vi "3d queue - Copia.vi"() -> ()   [LabVIEW 2020]
uses:
  control/Data Form.ctl
  control/file structure.ctl
  <vilib>/Analysis/1siggen.llb/Ramp Pattern by Samples.vi
  queue/Front Panel Message Queue.lvlib
  <vilib>/Analysis/NI_AALBase.lvlib
panel:
  out "XY Graph":cluster{"Ramp Pattern":dbl[], dbl[]}(graph)
  out "Data Loaded":dbl[][](array[numeric])
  out "Data Form":T1
  out "error out":errorcluster
  in  "error in":errorcluster
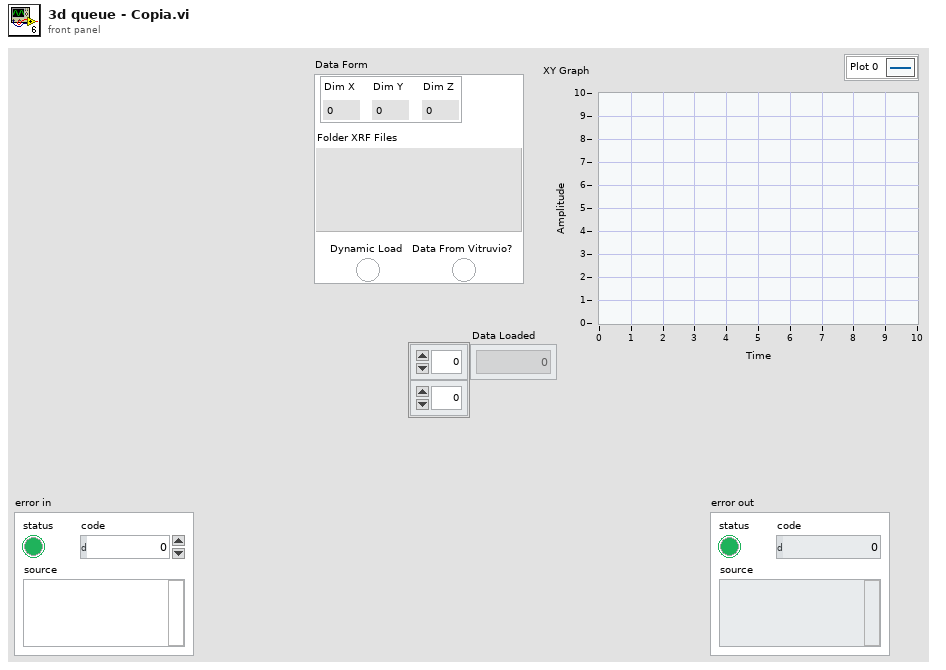
[diagram p1: front panel]
types:
  T1 = typedef "Data Form.ctl" = cluster{"Dimensions":cluster{"Dim X":i32, "Dim Y":i32, "Dim Z":i32}, "Folder XRF Files":path, "Dynamic Load":bool, "Data From Vitruvio?":bool}
  T2 = typedef "Front Panel Message Queue.lvlib/2d3d Message Queues.ctl" = cluster{"Main":refnum<queue>, "2d":refnum<queue>, "3d":refnum<queue>}
  T3 = typedef "file structure.ctl" = cluster{"Colonna":i32, "Offset Righe":i32, "Coda Righe":i32, "Transpose":bool}
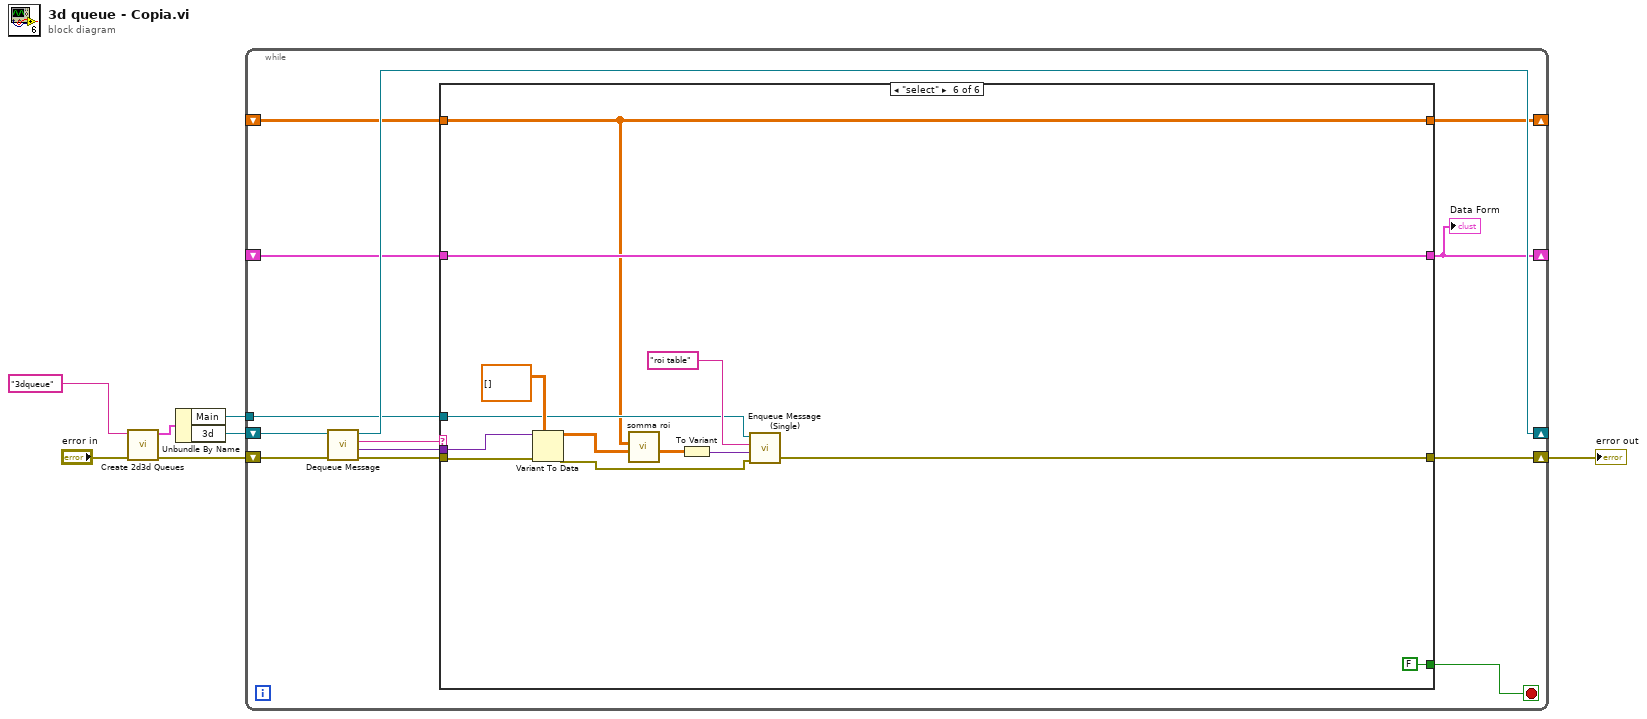
[diagram p0: block diagram]
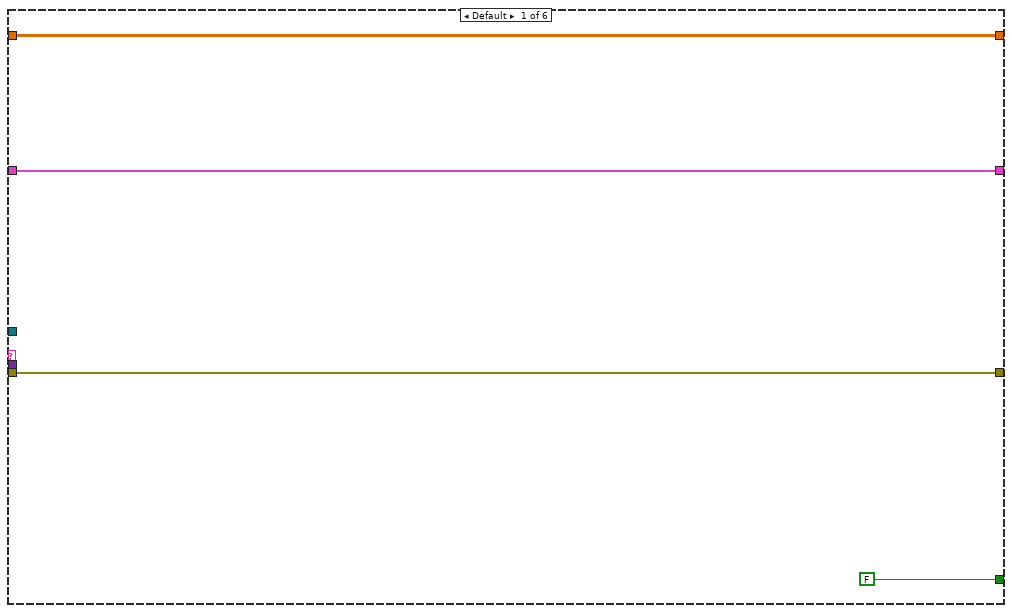
[diagram p2: hidden frame]
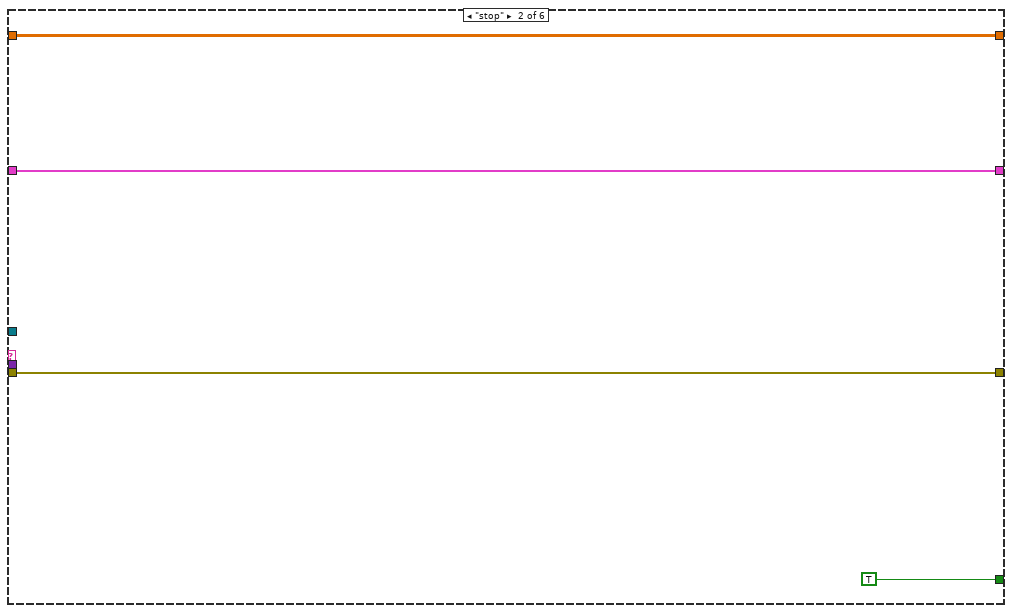
[diagram p3: hidden frame]
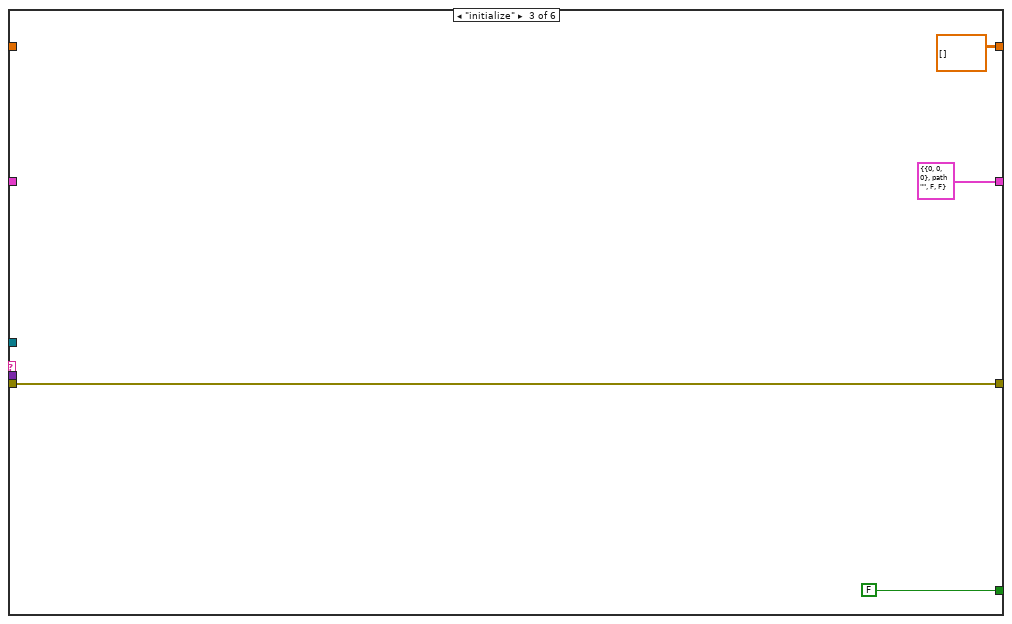
[diagram p4: hidden frame]
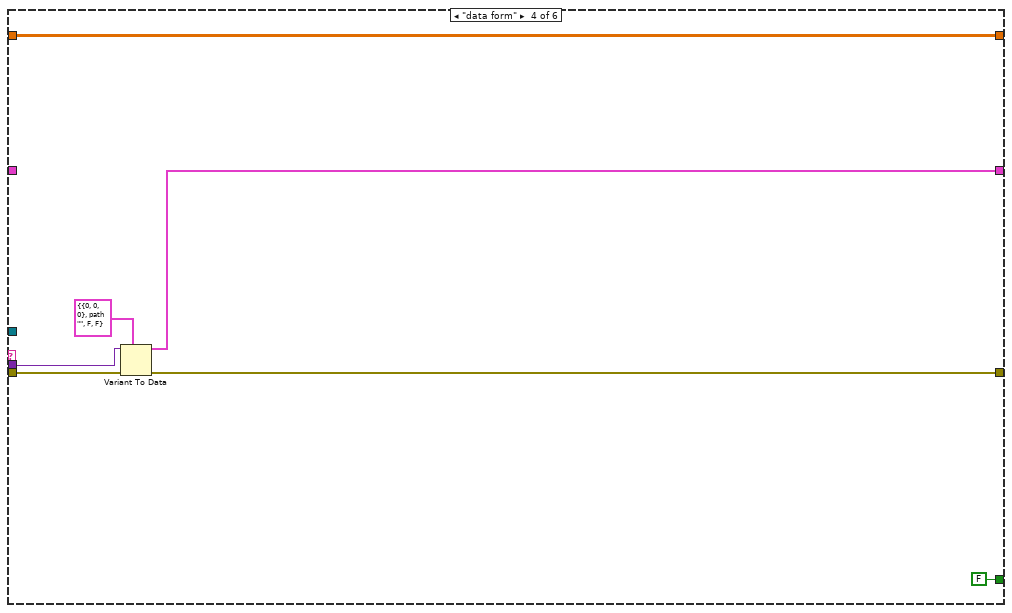
[diagram p5: hidden frame]
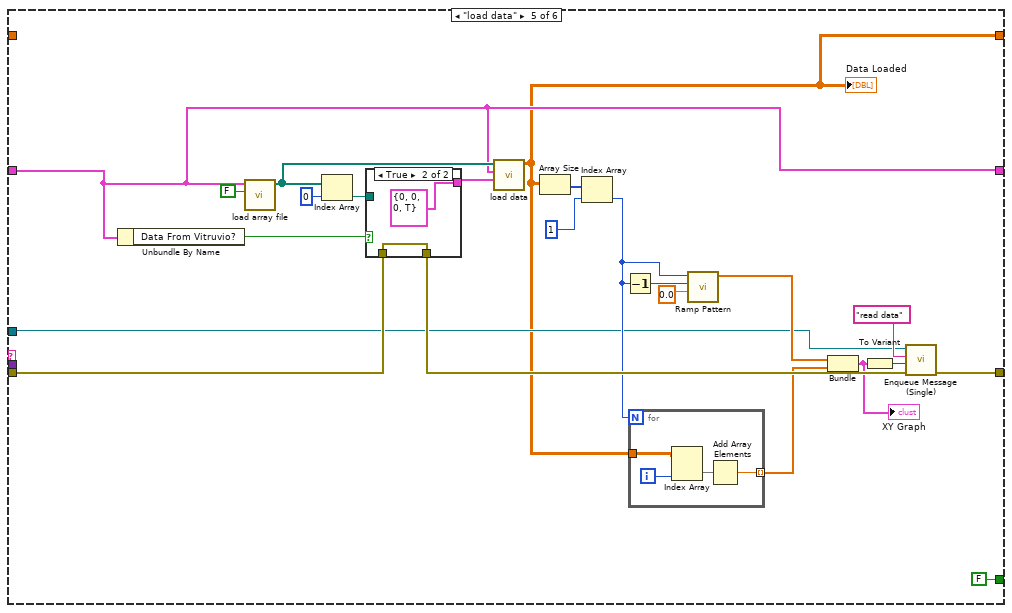
[diagram p6: hidden frame]
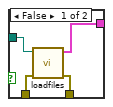
[diagram p7: hidden frame]
diagram:
  n1 = call "Create 2d3d Queues.vi"("error in (no error)"="error in", "name"="3dqueue") -> ("error out"=w3:errorcluster, "Message Queues"=w4:T2)  [unwired: 8 in]
  n2 = Unbundle By Name(w4) -> ("Main"=w1:refnum<queue>, "3d"=w7:refnum<queue>)
  n3 = while {
    shift-right: [w17] -> _
    shift-left: w7 -> [w19]
    shift-right: [w14] -> w6
    shift-left: w3 -> [w20]
    shift-right: [w12] -> _
    shift-left: _ -> [w13]
    shift-right: [w10] -> _
    shift-left: _ -> [w9]
    tunnel: w1 -> [w8]
    stop <- w15 stop-if-true
    n4 = call "Dequeue Message.vi"("error in (no error)"=w20, "Message Queue"=w19) -> ("error out"=w18:errorcluster, "Message Data"=w11:variant, "Message"=w16:string, "dup Message Queue"=w17:refnum<queue>)  [unwired: 5 in, 1 out]
    n5 = case shown="\"select\"" w16 {
      tunnel: w18 -> [w23 w27 w31 w37 w43 w80]
      tunnel: [FALSE TRUE FALSE FALSE FALSE FALSE] -> w15
      tunnel: [w23 w27 w31 w34 w44 w77] -> w14
      tunnel: [w22 w26 T1 {"Dimensions"={"Dim X"=0, "Dim Y"=0, "Dim Z"=0}, "Folder XRF Files"=path "", "Dynamic Load"=FALSE, "Data From Vitruvio?"=FALSE} ("Data Form") w35 w41 w78] -> w12
      tunnel: w13 -> [w22 w26 _ _ w41 w78]
      tunnel: w11 -> [_ _ _ w36 _ w79]
      tunnel: [w21 w25 dbl[][] [] ("Data Loaded") w33 w40 w73] -> w10
      tunnel: w9 -> [w21 w25 _ w33 _ w73]
      tunnel: w8 -> [_ _ _ _ w42 w81]
      frame Default {
      }
      frame "stop" {
      }
      frame "initialize" {
      }
      frame "data form" {
        n6 = Variant To Data(error in=w37, type=T1 {"Dimensions"={"Dim X"=0, "Dim Y"=0, "Dim Z"=0}, "Folder XRF Files"=path "", "Dynamic Load"=FALSE, "Data From Vitruvio?"=FALSE} ("Data Form"), Variant=w36) -> (data=w35:T1, error out=w34:errorcluster)
      }
      frame "load data" {
        n7 = Unbundle By Name(w41) -> ("Data From Vitruvio?"=w51:bool)
        n8 = call "load array file.vi"("2d?"=FALSE, "Data Form"=w41) -> ("File Array Out"=w58:path[])  [unwired: 9 in]
        n9 = Index Array(array=w58, index=0) -> (element=w59:path)
        n10 = case shown="True" w51 {
          tunnel: w59 -> [w64 _]
          tunnel: w43 -> [w66 w68]
          tunnel: [w63 T3 {"Colonna"=0, "Offset Righe"=0, "Coda Righe"=0, "Transpose"=TRUE} ("File Structure")] -> w57
          tunnel: [w65 w68] -> w54
          frame False {
            n11 = call "loadfiles.vi"("Error In"=w66, "First Spectrum"=w64) -> ("Error Out"=w65:errorcluster, "File Structure"=w63:T3)  [unwired: 8 in]
          }
          frame True {
          }
        }
        n12 = call "load data.vi"("File Structure"=w57, "Data Form"=w41, "File Array In"=w58) -> ("Data Loaded"=w40:dbl[][])  [unwired: 8 in]
        "Data Loaded" <- w40
        n13 = Array Size(array=w40) -> (size(s)=w56:i32[])
        n14 = Index Array(array=w56, index=1) -> (element=w48:i32)
        n15 = Decrement(x=w48) -> (x-1=w50:i32)
        n16 = for {
          N: w48 -> [_]
          tunnel: w40 -> [w71]
          tunnel: [w69] -> w46 mode=indexing
          i -> [w70]
          n17 = Index Array(array=w71, index (col)=w70) -> (element=w72:dbl[])  [unwired: 1 in]
          n18 = Add Array Elements(numeric array=w72) -> (sum=w69:dbl)
        }
        n19 = call-poly <vilib>:"Ramp Pattern.vi"("start"=0.0, "end"=w50, "samples"=w48) -> ("Ramp Pattern"=w47:dbl[])  [unwired: 7 in, 1 out]
        n20 = Bundle("Ramp Pattern"=w47, w46) -> (w45:cluster{"Ramp Pattern":dbl[], dbl[]})  [unwired: 1 in]
        "XY Graph" <- w45
        n21 = To Variant(anything=w45) -> (Variant=w52:variant)
        n22 = call "Enqueue Message (Single).vi"("error in (no error)"=w54, "Message Data"=w52, "Message"="read data", "Message Queue"=w42) -> ("error out"=w44:errorcluster)  [unwired: 6 in, 1 out]
      }
      frame "select" {
        n23 = Variant To Data(error in=w80, type=dbl[][] [] ("ROIs Min Max"), Variant=w79) -> (data=w74:dbl[][], error out=w83:errorcluster)
        n24 = call "somma roi.vi"("ROIs Min Max"=w74, "Data Loaded"=w73) -> ("ROIs Array Out"=w75:dbl[][])  [unwired: 9 in]
        n25 = To Variant(anything=w75) -> (Variant=w84:variant)
        n26 = call "Enqueue Message (Single).vi"("error in (no error)"=w83, "Message Data"=w84, "Message"="roi table", "Message Queue"=w81) -> ("error out"=w77:errorcluster)  [unwired: 6 in, 1 out]
      }
    }
    "Data Form" <- w12
  }
  "error out" <- w6
